vi "Send Email using SMTP Client Automated.vi"(8 "error in (no error)":errorcluster, 9 "Message":string, 10 "Subject":string, 11 "To:":string) -> ()   [LabVIEW 2019, in "GUI.lvlib"]
doc: "Uses the SMTP Email Client to send an email to a standard or secure SMTP server."
uses:
  GUI.lvlib
  <vilib>/smtpClient/SmtpClientHandle.ctl
  <vilib>/smtpClient/Set Message Text.vi
  <vilib>/smtpClient/LabVIEWSMTPClient.lvlib
panel:
  in  "Configure Server":bool
  in  "Sender's Email Address":string="cobrasysout@chromaus.com"
  in  "Password":string="Subzero2020"
  in  "Enable TLS":bool=TRUE
  in  "Username":string="cobrasysout@chromaus.com"
  in  "Port":string="587"
  in  "Outgoing Mail Server (SMTP)":string="smtp-mail.outlook.com"
  # "Overview: Connects to an SMTP Email Server, and sends one or more emails.\nRequirements: LabVIEW Full Development System\nInstructions:\n1. Run the VI.\n2. Configure the Outgoing Mail Server section, then click Configure Server.\n3. Specify the Compose Email content, then click Send Email.\n4. Click Stop to stop the VI."
  # "Outgoing Mail Server"
  # "Compose Email"
  # "Optional Parameters"
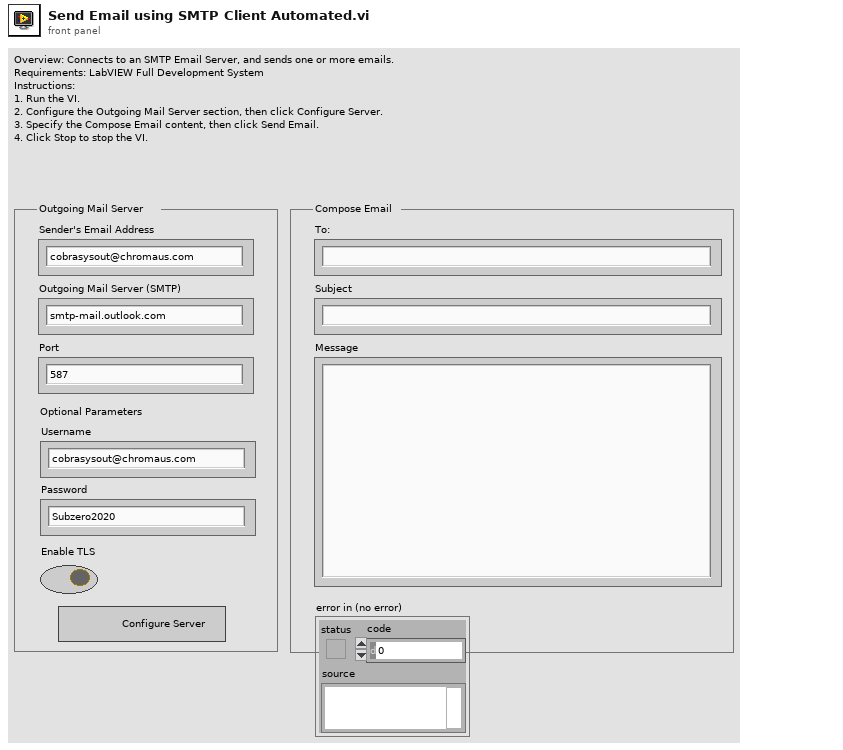
[diagram p1: front panel]
types:
  T1 = typedef "LabVIEWSMTPClient.lvlib/SmtpClientHandle.ctl" = refnum<k1>
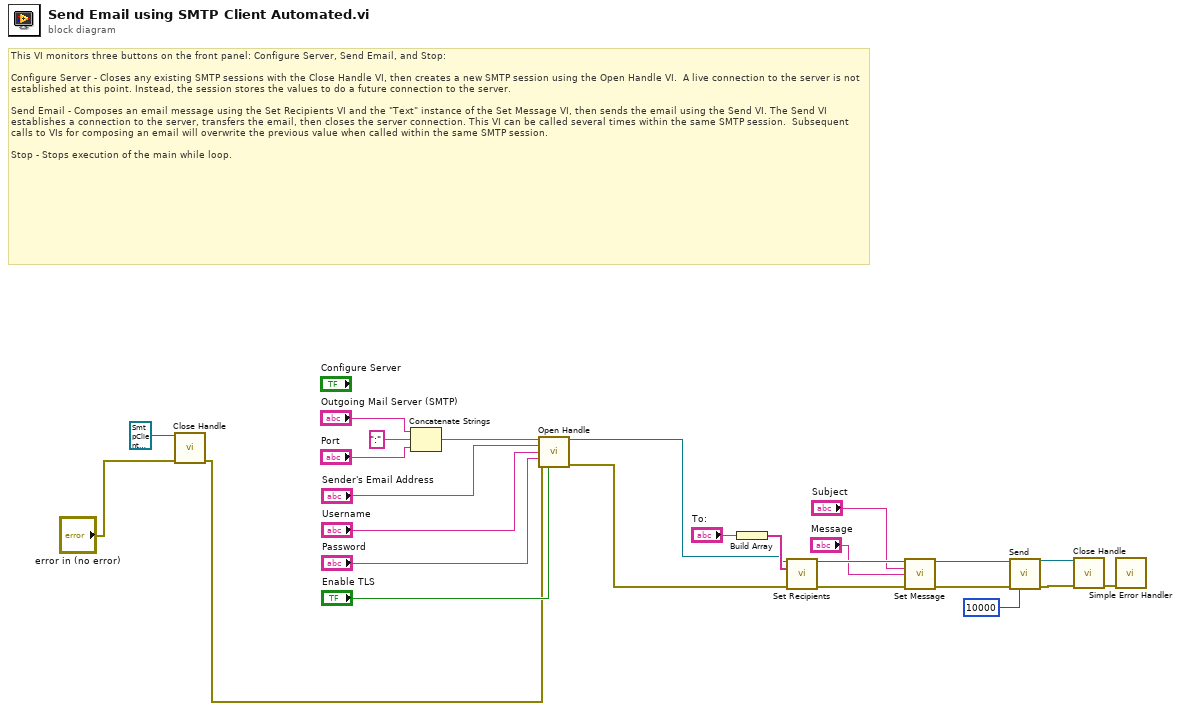
[diagram p0: block diagram]
diagram:
  # "This VI monitors three buttons on the front panel: Configure Server, Send Email, and Stop:\n\nConfigure Server - Closes any existing SMTP sessions with the Close Handle VI, then creates a new SMTP session using the Open Handle VI.  A live connection to the server is not established at this point. Instead, the session stores the values to do a future connection to the server.\n\nSend Email - Composes an email message using the Set Recipients VI and the \"Text\" instance of the Set Message VI, then sends the email using the Send VI. The Send VI establishes a connection to the server, transfers the email, then closes the server connection. This VI can be called several times within the same SMTP session.  Subsequent calls to VIs for composing an email will overwrite the previous value when called within the same SMTP session.\n\nStop - Stops execution of the main while loop."
  n1 = call <vilib>:"Close Handle.vi"("handle in"=T1 refnum ("handle out"), "error in (no error)"="error in (no error)") -> ("error out"=w2:errorcluster)  [unwired: 12 in, 1 out]
  n2 = Concatenate Strings("Outgoing Mail Server (SMTP)", ":" ("string"), "Port") -> (w8:string)
  n3 = call <vilib>:"Open Handle.vi"("server address"=w8, "from"="Sender's Email Address", "username"="Username", "password"="Password", "error in (no error)"=w2, "use TLS (false)"="Enable TLS") -> ("handle out"=w4:T1, "error out"=w1:errorcluster)  [unwired: 8 in]
  n4 = Build Array("To:") -> (w17:string[])
  n5 = call <vilib>:"Set Recipients.vi"("handle in"=w4, "to"=w17, "error in (no error)"=w1) -> ("handle out"=w21:T1, "error out"=w18:errorcluster)  [unwired: 11 in]
  n6 = call-poly <vilib>:"Set Message.vi"("handle in"=w21, "subject"="Subject", "plain text message"="Message", "error in (no error)"=w18) -> ("handle out"=w23:T1, "error out"=w22:errorcluster)  [unwired: 10 in]
  n7 = call <vilib>:"Send.vi"("handle in"=w23, "error in (no error)"=w22, "timeout in ms (10000)"=10000 ("timeout in ms")) -> ("handle out"=w14:T1, "error out"=w13:errorcluster)  [unwired: 10 in, 1 out]
  n8 = call <vilib>:"Close Handle.vi"("handle in"=w14, "error in (no error)"=w13) -> ("error out"=w24:errorcluster)  [unwired: 12 in, 1 out]
  n9 = call <vilib>:"Simple Error Handler.vi"("error in (no error)"=w24) -> ()  [unwired: 4 in, 5 out]
